vi "LWXPS_TCLScriptExecute.vi"(0 "XPS Reference IN":refnum<k24>, 5 "TCL File Name":string, 7 "Task Name":string, 9 "Parameter List":string, 11 "LabVIEW error IN":errorcluster) -> (4 "XPS Reference OUT":refnum<k24>, 6 "Returned error code":i32, 8 "XPS Error String":string, 15 "LabVIEW error OUT":errorcluster)   [LabVIEW 2014]
uses:
  D:/XPSQ8_LabView_Library/Development/Source/Dll/Newport.XPS.CommandInterface.dll
  Dll/Newport.XPS.CommandInterface.dll
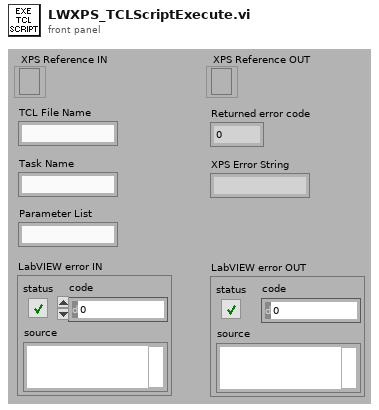
[diagram p1: front panel]
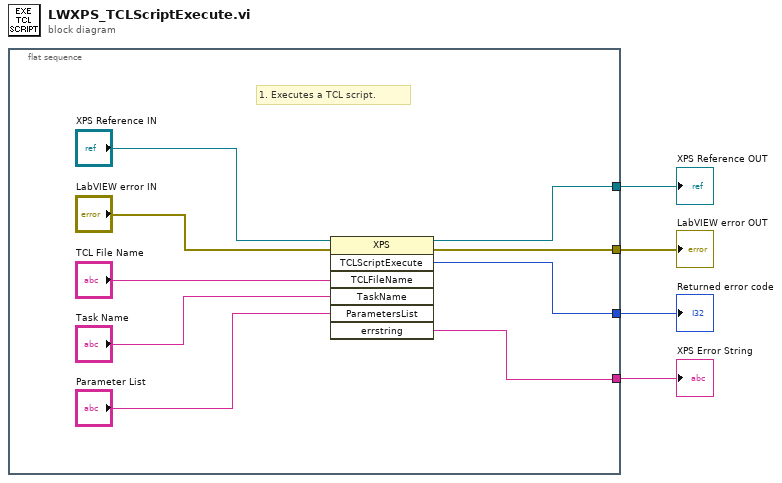
[diagram p0: block diagram]
diagram:
  n1 = flat-sequence {
    tunnel: [w9] -> w4
    tunnel: [w8] -> w3
    tunnel: [w10] -> w2
    tunnel: [w7] -> w1
    frame #0 {
      # "1. Executes a TCL script."
      n2 = invoke class="XPS" method="TCLScriptExecute"(reference="XPS Reference IN", error in="LabVIEW error IN", "TCLFileName"="TCL File Name", "TaskName"="Task Name", "ParametersList"="Parameter List") -> (reference out=w9:refnum<k24>, error out=w8:errorcluster, "TCLScriptExecute"=w10:i32, "errstring"=w7:string)  [unwired: 2 in, 3 out]
    }
  }
  "XPS Error String" <- w1
  "XPS Reference OUT" <- w4
  "LabVIEW error OUT" <- w3
  "Returned error code" <- w2
